vi "take and write data.vi"(9 "y":dbl, 10 "Path":path, 11 "Current position (units)":dbl) -> ()   [LabVIEW 2011]
uses:
  <vilib>/Utility/file.llb/Write To Spreadsheet File (DBL).vi
panel:
  out "array":i32[](array[numeric])
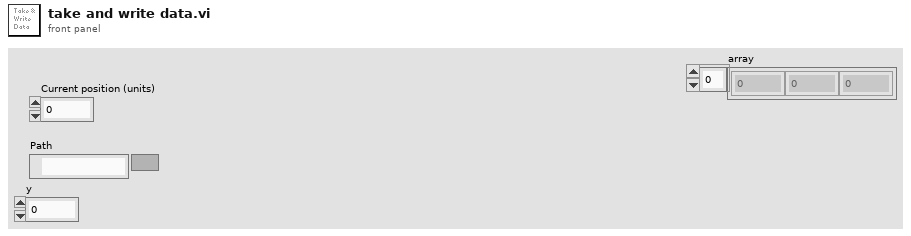
[diagram p1: front panel]
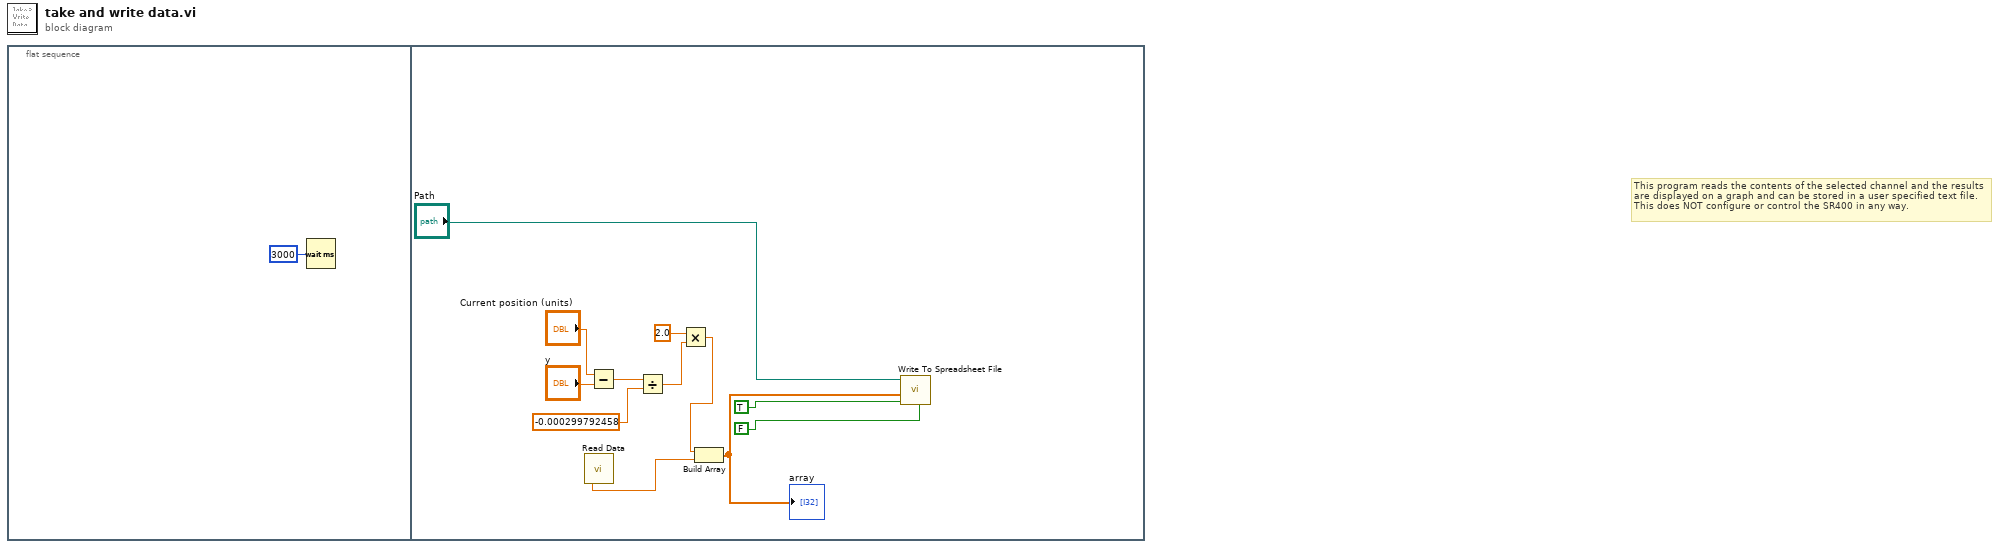
[diagram p0: block diagram]
diagram:
  # "This program reads the contents of the selected channel and the results\nare displayed on a graph and can be stored in a user specified text file.\nThis does NOT configure or control the SR400 in any way."
  n1 = flat-sequence {
    frame #0 {
      n2 = Wait (ms)(milliseconds to wait=u32 3000) -> ()  [unwired: 1 out]
    }
    frame #1 {
      n3 = call "Read Data.vi"() -> ("data"=w6:dbl)  [unwired: 3 in]
      n4 = Subtract(x="Current position (units)", y="y") -> (x-y=w8:dbl)
      n5 = Divide(x=w8, y=-0.000299792458) -> (x/y=w4:dbl)
      n6 = Multiply(x=2.0, y=w4) -> (x*y=w3:dbl)
      n7 = Build Array(w3, w6) -> (w5:dbl[])
      "array" <- w5
      n8 = call-poly <vilib>:"Write To Spreadsheet File.vi"("transpose? (no:F)"=FALSE, "append to file? (new file:F)"=TRUE, "1D data"=w5, "file path (dialog if empty)"="Path") -> ()  [unwired: 4 in, 1 out]
    }
  }
